vi "test_generator.vi"() -> ()   [LabVIEW 2020]
panel:
  out "XY Graph":cluster{"X":dbl, "Y":dbl}[](graph)
  out "Plan":string
  in  "Accel length":dbl
  in  "Segments per side":i32
  in  "Radius":dbl
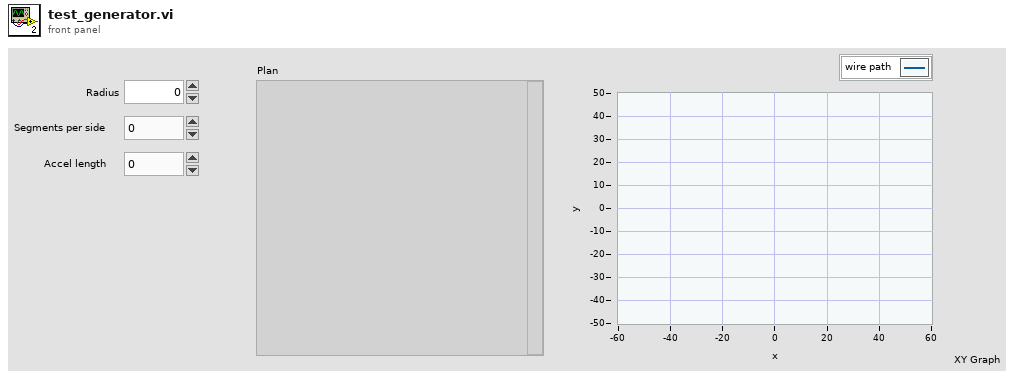
[diagram p1: front panel]
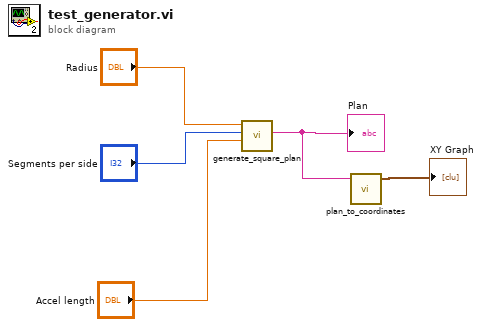
[diagram p0: block diagram]
diagram:
  n1 = call "generate_square_plan.vi"("Accel length"="Accel length", "Segments per side"="Segments per side", "Radius"="Radius") -> ("Plan"=w2:string)  [unwired: 3 in, 1 out]
  "Plan" <- w2
  n2 = call "plan_to_coordinates.vi"("Plan GCode"=w2) -> ("XY Graph"=→"XY Graph":cluster{"X":dbl, "Y":dbl}[])  [unwired: 3 in, 1 out]
